vi "AMC e.bloxx Write Value - Boolean.vi"(6 "Value":bool, 8 "error in (no error)":errorcluster, 9 "Channel":i32, 10 "Module Address":i32, 11 "VISA Resource Name":refnum<visa-resource-name>) -> (0 "error out":errorcluster, 3 "VISA Resource Name out":refnum<visa-resource-name>)   [LabVIEW 2013]
doc: "<B>AMC - Analytik & Messtechnik GmbH Chemnitz</B>\n\nLabVIEW Drivers for e.bloxx series from Gantner Instruments\n\nThis VI writes a value to a variable specified by <B>Module Address</B> and <B>Variable</B> (starts counting with 0)."
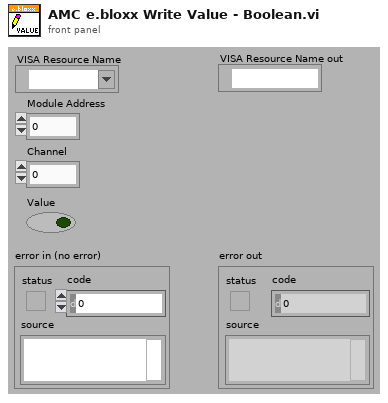
[diagram p1: front panel]
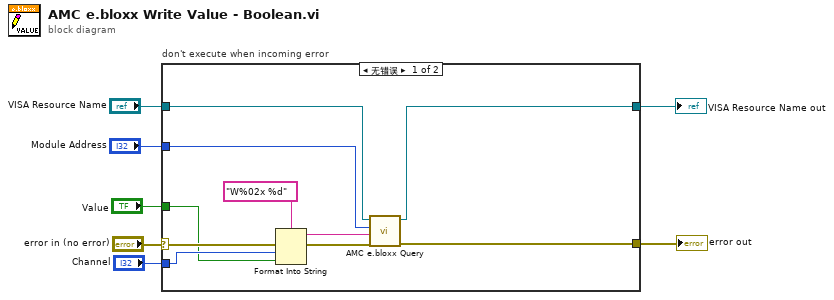
[diagram p0: block diagram]
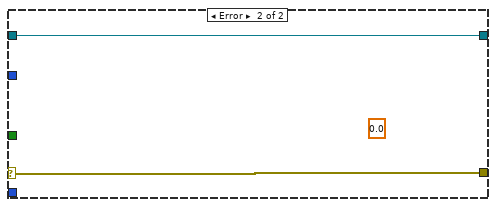
[diagram p2: hidden frame]
diagram:
  n1 = case "don't execute when incoming error" shown="无错误" "error in (no error)" {
    selector: "error in (no error)" -> [w14 w19]
    tunnel: [w8 w19] -> w6
    tunnel: "VISA Resource Name" -> [w16 w18]
    tunnel: "Module Address" -> [w17 _]
    tunnel: [w15 w18] -> w3
    tunnel: "Channel" -> [w12 _]
    tunnel: "Value" -> [w9 _]
    frame No Error {
      n2 = Format Into String(format string="W%02x %d", error in=w14, w12, w9) -> (resulting string=w11:string, error out=w13:errorcluster)  [unwired: 1 in]
      n3 = call "AMC e.bloxx Query.vi"("error in (no error)"=w13, "Module Command"=w11, "Module Address"=w17, "VISA Resource Name"=w16) -> ("error out"=w8:errorcluster, "VISA Resource Name out"=w15:refnum<visa-resource-name>)  [unwired: 5 in, 1 out]
    }
    frame Error {
      (unwired) 0.0
    }
  }
  "error out" <- w6
  "VISA Resource Name out" <- w3
